vi "derivative.vi"(8 "Reset":bool, 10 "Starting value":dbl, 11 "x":dbl) -> (3 "dx/dt":dbl)   [LabVIEW 2020]
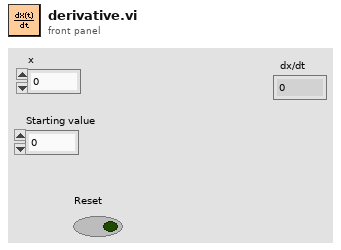
[diagram p1: front panel]
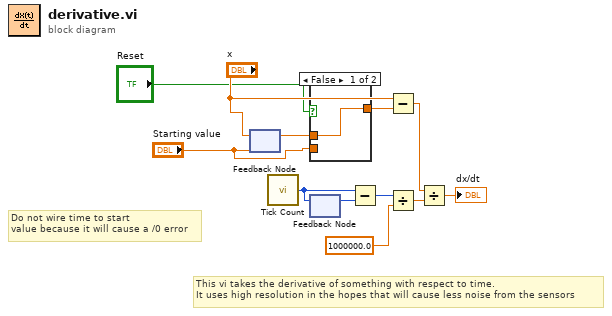
[diagram p0: block diagram]
diagram:
  # "Do not wire time to start\nvalue because it will cause a /0 error"
  # "This vi takes the derivative of something with respect to time.\nIt uses high resolution in the hopes that will cause less noise from the sensors"
  n1 = feedback #1("Starting value") -> (w1:dbl)
  n2 = feedback-in #1("x") -> ()
  n3 = call "Tick Count"() -> ("Tick Count(uSec)"=w5:u32)
  n4 = case shown="False" "Reset" {
    tunnel: "Starting value" -> [_ w14]
    tunnel: [w13 w14] -> w2
    tunnel: w1 -> [w13 _]
    frame False {
    }
    frame True {
    }
  }
  n5 = feedback #2() -> (w10:u32)  [unwired: 1 in]
  n6 = feedback-in #2(w5) -> ()
  n7 = Subtract(x=w5, y=w10) -> (x-y=w8:u32)
  n8 = Subtract(x="x", y=w2) -> (x-y=w11:dbl)
  n9 = Divide(x=w8, y=1000000.0) -> (x/y=w6:dbl)
  n10 = Divide(x=w11, y=w6) -> (x/y=→"dx/dt":dbl)
